vi "Is Public.vi"(11 "ProjectItem Refnum":refnum<vi>) -> (2 "Is Public":bool)   [LabVIEW 2017, in "LVUnit Test Discoverer.lvclass"]
uses:
  LVUnit Test Discoverer.lvclass
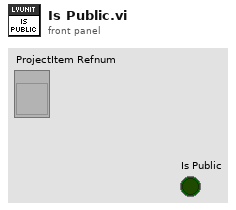
[diagram p1: front panel]
types:
  T1 = enum32{"invalid scope", "public", "private", "protected", "community"}
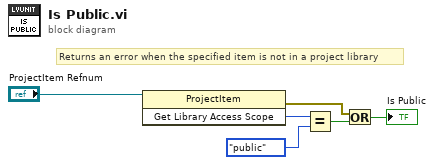
[diagram p0: block diagram]
diagram:
  # "Returns an error when the specified item is not in a project library"
  n1 = invoke class="ProjectItem" method="Get Library Access Scope"(reference="ProjectItem Refnum") -> (error out=w2:errorcluster, "Get Library Access Scope"=w6:T1)  [unwired: 2 in, 1 out]
  n2 = Equal?(x=w6, y=T1."public") -> (x = y?=w3:bool)
  n3 = Or(x=w2, y=w3) -> (x .or. y?=→"Is Public":bool)
